vi "Read Limit File.vi"(7 "base path":path=path "C:/Users/user/Documents/AD2255/limits", 11 "FIle_Name":string="KGD_Limit_File") -> (3 "Master_Limits_Info":string[][](array[string])=[["Test Number", "Generic Test Name\n", "Variant", "HV_Trim_Settings\n", "Low Limit\n", "High Limit\n"], ["100", "test1", "26", "10,11,12,13", "10", "20"], ["103", "est2", "29", "31,30,0,21", "30", "40"]])   [LabVIEW 2013]
uses:
  <vilib>/Utility/file.llb/Read From Spreadsheet File (string).vi
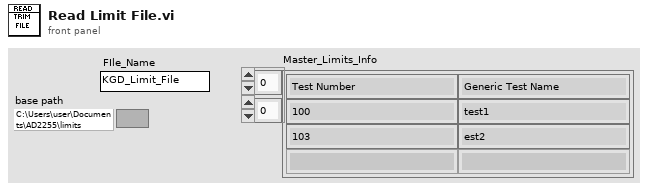
[diagram p1: front panel]
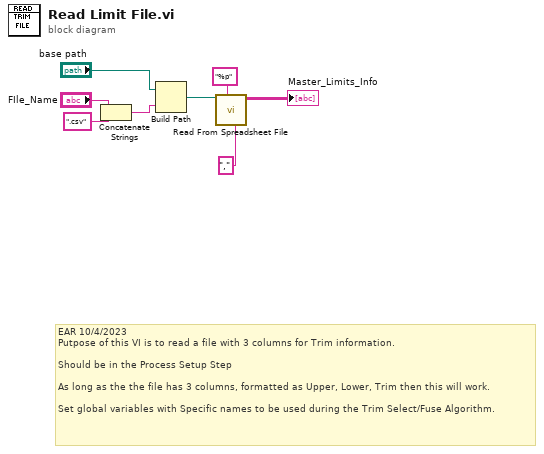
[diagram p0: block diagram]
diagram:
  # "EAR 10/4/2023\nPutpose of this VI is to read a file with 3 columns for Trim information.\n\nShould be in the Process Setup Step\n\nAs long as the the file has 3 columns, formatted as Upper, Lower, Trim then this will work.\n\nSet global variables with Specific names to be used during the Trim Select/Fuse Algorithm."
  n1 = Concatenate Strings("FIle_Name", ".csv" ("string")) -> (w6:string)
  n2 = Build Path(base path="base path", name or relative path=w6) -> (appended path=w5:path)
  n3 = call-poly <vilib>:"Read From Spreadsheet File.vi"("delimiter (\\t)"="," ("delimiter (\\t)"), "format (%s)"="%p", "file path (dialog if empty)"=w5) -> ("all rows"=→"Master_Limits_Info":string[][])  [unwired: 4 in, 4 out]
